vi "Stop Core.vi"(10 "final error code":i32 caption="最终错误代码", 11 "工况数据UI in":refnum<class "工况数据UI.lvclass"> caption="操作者输入") -> (3 "工况数据UI out":refnum<class "工况数据UI.lvclass"> caption="操作者输出")   [LabVIEW 2016, in "工况数据UI.lvlib" / "工况数据UI.lvclass"]
doc: "(<B>Filename</B>: Actor Framework.lvlib:Actor.lvclass:Stop Core.vi)\n\nDefines what the actor does before it stops. Use the <B>final error code</B> input to determine whether the actor shut down in response to an error.\n\nBy default, this method does nothing.子孙类重写该方法，定义出错时的操作，例如，关闭操作者核心方法初始的进程。"
uses:
  <vilib>/ActorFramework/Actor/Actor.lvclass
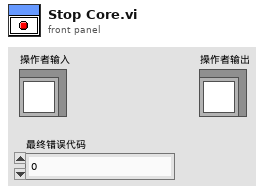
[diagram p1: front panel]
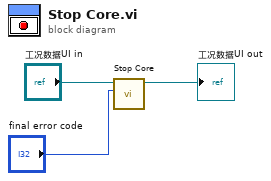
[diagram p0: block diagram]
diagram:
  n1 = call-parent "Stop Core.vi"("final error code"="final error code", "Actor in"="工况数据UI in") -> ("Actor out"=→"工况数据UI out":refnum<class "工况数据UI.lvclass">)  [unwired: 9 in]
